vi "chaos_crest_get.vi"(0 "cuname":string, 1 "cmd":string, 2 "args":string, 3 "timeout (10000)":i32=10000, 4 "handleConnection":T2, 7 "prio":i32=50, 8 "sched (ms)":i32=100, 9 "cmd submission mode":enum16{"stack", "kill previous"}(ring)) -> (5 "body":string, 6 "headers":string, 10 "nok":i32)   [LabVIEW 2014, in "chaosui-crest.lvlib"]
uses:
  chaosui-crest.lvlib
  <vilib>/httpClient/ClientHandle.ctl
  <vilib>/httpClient/LabVIEWHTTPClient.lvlib
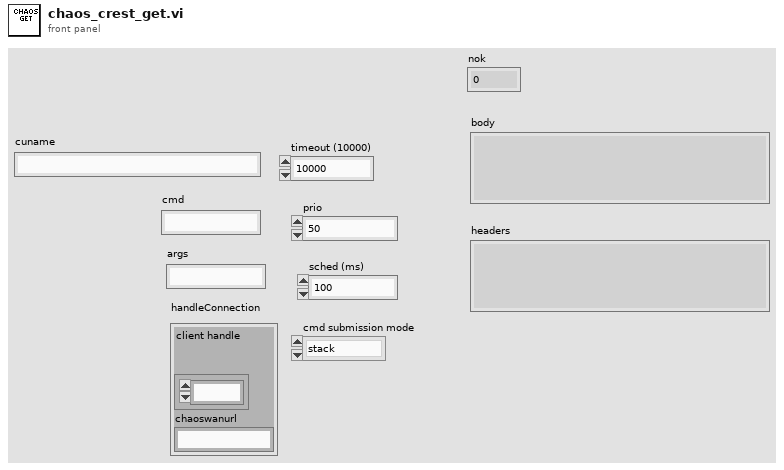
[diagram p1: front panel]
types:
  T1 = typedef "LabVIEWHTTPClient.lvlib/ClientHandle.ctl" = refnum<k1>
  T2 = cluster{"client handle":T1, "chaoswanurl":string}
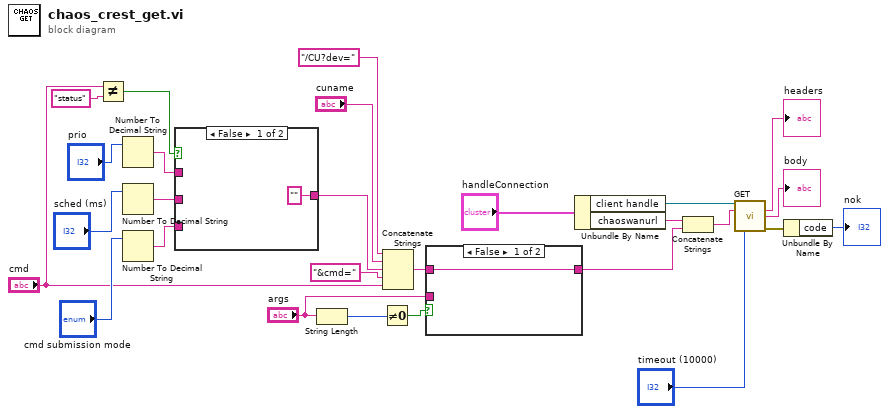
[diagram p0: block diagram]
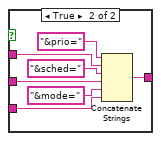
[diagram p2: hidden frame]
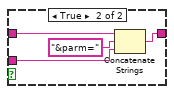
[diagram p3: hidden frame]
diagram:
  n1 = Not Equal?(x="cmd", y="status") -> (x != y?=w4:bool)
  n2 = Number To Decimal String(number="prio") -> (decimal integer string=w8:string)  [unwired: 1 in]
  n3 = Number To Decimal String(number="sched (ms)") -> (decimal integer string=w7:string)  [unwired: 1 in]
  n4 = Number To Decimal String(number="cmd submission mode") -> (decimal integer string=w6:string)  [unwired: 1 in]
  n5 = case shown="False" w4 {
    tunnel: w8 -> [_ w34]
    tunnel: w7 -> [_ w32]
    tunnel: w6 -> [_ w30]
    tunnel: ["" w29] -> w1
    frame False {
    }
    frame True {
      n6 = Concatenate Strings("&prio=", w34, "&sched=", w32, "&mode=", w30) -> (w29:string)
    }
  }
  n7 = String Length(string="args") -> (length=w23:i32)
  n8 = Not Equal To 0?(x=w23) -> (x != 0?=w22:bool)
  n9 = Concatenate Strings("/CU?dev=" ("string"), "cuname", w1, "&cmd=" ("string"), "cmd") -> (w21:string)
  n10 = case shown="False" w22 {
    tunnel: w21 -> [w36 w40]
    tunnel: "args" -> [_ w38]
    tunnel: [w36 w37] -> w19
    frame False {
    }
    frame True {
      n11 = Concatenate Strings(w40, "&parm=" ("string"), w38) -> (w37:string)
    }
  }
  n12 = Unbundle By Name("handleConnection") -> ("client handle"=w18:T1, "chaoswanurl"=w26:string)
  n13 = Concatenate Strings(w26, w19) -> (w17:string)
  n14 = call <vilib>:"GET.vi"("client handle"=w18, "url"=w17, "timeout (10000)"="timeout (10000)") -> ("headers"=→"headers":string, "body"=→"body":string, "error out"=w16:errorcluster)  [unwired: 9 in, 1 out]
  n15 = Unbundle By Name(w16) -> ("code"=→"nok":i32)
